vi "gateway设置.vi"() -> ()   [LabVIEW 2012]
panel:
  out "写入缓冲区":string
  out "制热":bool
  out "制冷":bool
  in  "确定按钮":bool
  in  "环境设定":enum16{"不做控制", "清凉夏日", "温暖冬日", "自定义"}(ring)
  in  "亮度阈值":i32
  in  "温度阈值":i32
  in  "电源阈值":dbl min=0.0 max=5.0
  # "自定义"
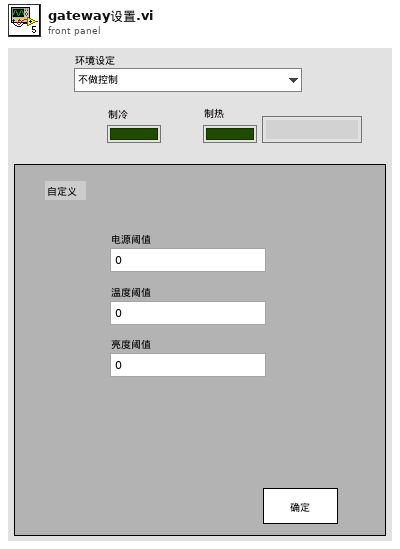
[diagram p1: front panel]
types:
  T1 = cluster{i32, enum16{"温度", "亮度", "电量", "连接质量"}, sgl}
  T2 = enum8{"Enabled", "Disabled", "Disabled and Grayed Out"}
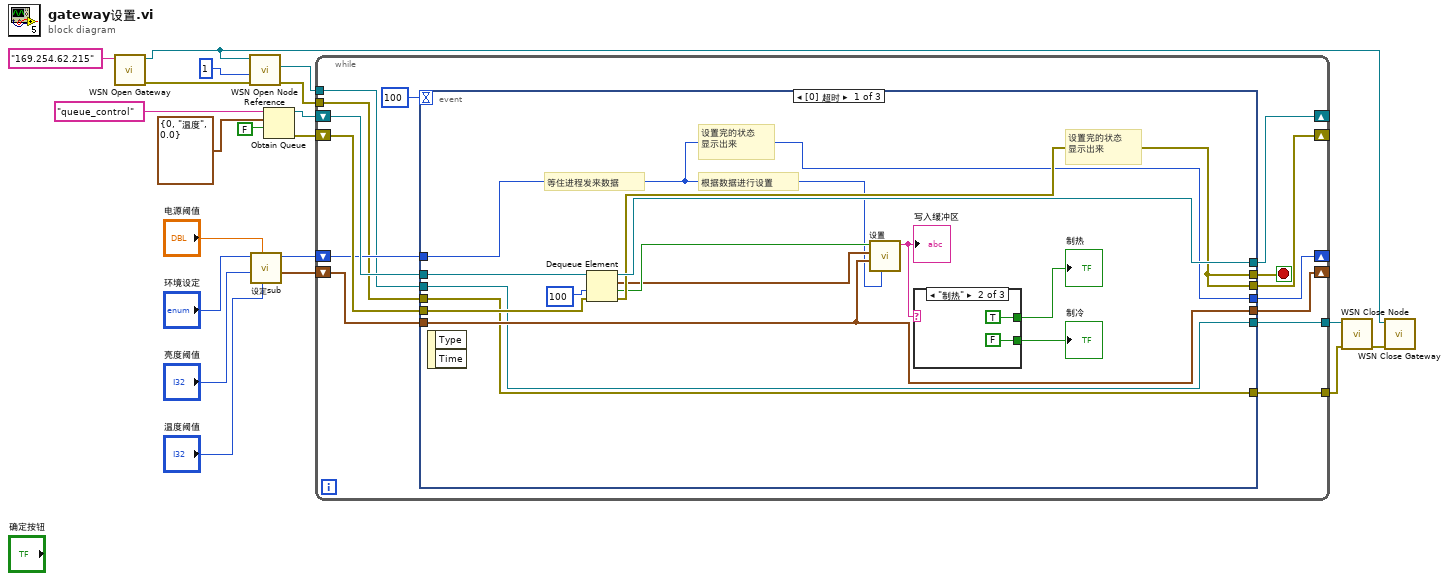
[diagram p0: block diagram]
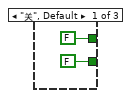
[diagram p2: hidden frame]
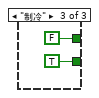
[diagram p3: hidden frame]
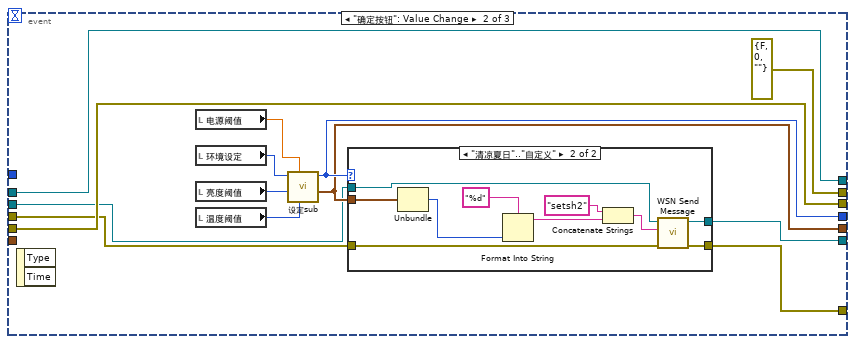
[diagram p4: hidden frame]
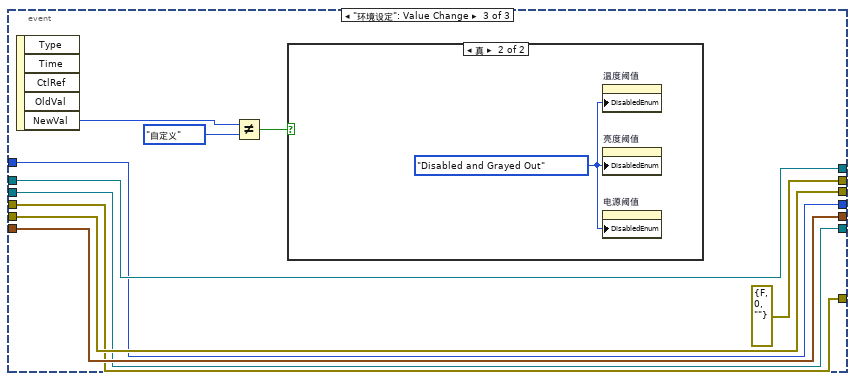
[diagram p6: hidden frame]
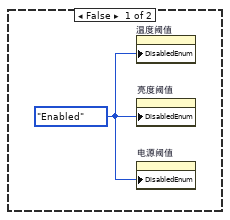
[diagram p7: hidden frame]
diagram:
  n1 = call <vilib>:"WSN Open Gateway.vi"("IP address"="169.254.62.215") -> ("error out"=w15:errorcluster, "gateway reference"=w2:refnum<k20>)  [unwired: 9 in]
  n2 = call <vilib>:"WSN Open Node Reference.vi"("error in (no error)"=w15, "ID"=u32 1, "gateway reference"=w2) -> ("error out"=w12:errorcluster, "node reference"=w13:refnum<k20>)  [unwired: 6 in, 1 out]
  n3 = call "设定sub.vi"("温度阈值"="温度阈值", "电源阈值"="电源阈值", "亮度阈值"="亮度阈值", "环境设定"="环境设定") -> ("输出簇"=w7:cluster{"温度阈值":i32, "亮度阈值":i32, "电源阈值":dbl}, "环境设定out"=w6:enum16{"不做控制", "清凉夏日", "温暖冬日", "自定义"})  [unwired: 5 in]
  n4 = Obtain Queue(name (unnamed)="queue_control" ("名称（未命名）"), element data type=T1 {0, enum."温度", 0.0}, create if not found? (T)=FALSE ("如未找到是否创建？(T)")) -> (queue out=w1:refnum<queue>, error out=w19:errorcluster)  [unwired: 2 in, 1 out]
  n5 = while {
    shift-right: [w31] -> _
    shift-left: w1 -> [w33]
    shift-right: [w30] -> _
    shift-left: w19 -> [w32]
    shift-right: [w28] -> _
    shift-left: w6 -> [w25]
    tunnel: w13 -> [w24]
    tunnel: w12 -> [w23]
    shift-right: [w27] -> _
    shift-left: w7 -> [w26]
    tunnel: [w22] -> w5
    tunnel: [w21] -> w4
    stop <- w34 stop-if-true
    n6 = event shown="[0] 超时" {
      selector: _ -> [_ _ _]
      dyn-events: _ -> [_ _ _]
      timeout: 100 -> [_ _ _]
      tunnel: [w45 errorcluster {"status"=FALSE, "code"=0, "source"=""} ("error out") errorcluster {"status"=FALSE, "code"=0, "source"=""} ("error out")] -> w34
      tunnel: w33 -> [w48 w63 w87]
      tunnel: w32 -> [w47 w64 w86]
      tunnel: [w46 w63 w87] -> w31
      tunnel: [w45 w64 w86] -> w30
      tunnel: [w40 w60 w82] -> w28
      tunnel: [w41 w59 w83] -> w27
      tunnel: w26 -> [w41 _ w83]
      tunnel: w25 -> [w40 _ w82]
      tunnel: w24 -> [w38 w58 w80]
      tunnel: w23 -> [w39 w57 w81]
      tunnel: [w39 w55 w81] -> w22
      tunnel: [w38 w56 w80] -> w21
      event Timeout {
        # "设置完的状态\n显示出来"
        # "设置完的状态\n显示出来"
        # "根据数据进行设置"
        # "等住进程发来数据"
        n7 = event-data() -> ()  [unwired: 1 in, 2 out]
        n8 = Dequeue Element(queue=w48, timeout in ms (-1)=100 ("超时毫秒(-1)"), error in (no error)=w47) -> (queue out=w46:refnum<queue>, element=w43:T1, timed out?=w44:bool, error out=w45:errorcluster)
        n9 = call "设置.vi"("环境设定out"=w40, "输出数值"=w41, "消息"=w43, "timed out?"=w44) -> ("写入缓冲区"=w37:string)  [unwired: 7 in]
        "写入缓冲区" <- w37
        n10 = case shown="\"制热\"" w37 {
          tunnel: [FALSE FALSE TRUE] -> w36
          tunnel: [FALSE TRUE FALSE] -> w35
          frame "关", Default {
          }
          frame "制热" {
          }
          frame "制冷" {
          }
        }
        "制冷" <- w36
        "制热" <- w35
      }
      event "确定按钮": Value Change {
        n11 = event-data() -> ()  [unwired: 1 in, 2 out]
        n12 = local read "电源阈值"() -> (w65:dbl)
        n13 = local read "环境设定"() -> (w61:enum16{"不做控制", "清凉夏日", "温暖冬日", "自定义"})
        n14 = local read "亮度阈值"() -> (w67:i32)
        n15 = local read "温度阈值"() -> (w66:i32)
        n16 = call "设定sub.vi"("温度阈值"=w66, "电源阈值"=w65, "亮度阈值"=w67, "环境设定"=w61) -> ("输出簇"=w59:cluster{"温度阈值":i32, "亮度阈值":i32, "电源阈值":dbl}, "环境设定out"=w60:enum16{"不做控制", "清凉夏日", "温暖冬日", "自定义"})  [unwired: 5 in]
        n17 = case shown="\"清凉夏日\"..\"自定义\"" w60 {
          tunnel: w59 -> [_ w79]
          tunnel: w58 -> [w69 w73]
          tunnel: w57 -> [w68 w72]
          tunnel: [w69 w71] -> w56
          tunnel: [w68 w70] -> w55
          frame "不做控制", Default {
          }
          frame "清凉夏日".."自定义" {
            n18 = Unbundle(w79) -> ("亮度阈值"=w78:i32)  [unwired: 2 out]
            n19 = Format Into String(format string="%d" ("格式字符串"), w78) -> (resulting string=w76:string)  [unwired: 2 in, 1 out]
            n20 = Concatenate Strings("setsh2", w76) -> (w74:string)
            n21 = call <vilib>:"WSN Send Message.vi"("error in (no error)"=w72, "message"=w74, "node reference"=w73) -> ("error out"=w70:errorcluster, "node reference"=w71:refnum<k20>)  [unwired: 6 in, 1 out]
          }
        }
      }
      event "环境设定": Value Change {
        n22 = event-data() -> ("NewVal"=w88:enum16{"不做控制", "清凉夏日", "温暖冬日", "自定义"})  [unwired: 1 in, 4 out]
        n23 = Not Equal?(x=w88, y=enum16{"不做控制", "清凉夏日", "温暖冬日", "自定义"}."自定义" ("环境设定")) -> (x != y?=w89:bool)
        n24 = case shown="真" w89 {
          frame False {
            w90 = T2."Enabled" ("禁用")
            n25 = property on="温度阈值" class="DigNum (严格)"("DisabledEnum"=w90) -> ()  [unwired: 2 in, 2 out]
            n26 = property on="亮度阈值" class="DigNum (严格)"("DisabledEnum"=w90) -> ()  [unwired: 2 in, 2 out]
            n27 = property on="电源阈值" class="DigNum (严格)"("DisabledEnum"=w90) -> ()  [unwired: 2 in, 2 out]
          }
          frame True {
            w91 = T2."Disabled and Grayed Out" ("禁用")
            n28 = property on="温度阈值" class="DigNum (严格)"("DisabledEnum"=w91) -> ()  [unwired: 2 in, 2 out]
            n29 = property on="亮度阈值" class="DigNum (严格)"("DisabledEnum"=w91) -> ()  [unwired: 2 in, 2 out]
            n30 = property on="电源阈值" class="DigNum (严格)"("DisabledEnum"=w91) -> ()  [unwired: 2 in, 2 out]
          }
        }
      }
    }
  }
  n31 = call <vilib>:"WSN Close Node.vi"("error in (no error)"=w5, "node reference"=w4) -> ("error out"=w3:errorcluster)  [unwired: 9 in]
  n32 = call <vilib>:"WSN Close Gateway.vi"("error in (no error)"=w3, "gateway reference"=w2) -> ()  [unwired: 9 in, 1 out]
